vi "Demo.vi"(0 "LED Outputs":T4, 1 "VISA resource name":refnum<visa-resource-name>="COM5", 2 "Stop":bool) -> (14 "Analog Inputs":T2, 15 "Switch Inputs":T3, 16 "Updates / Second":dbl, 17 "CRC Status":bool, 18 "CRC Failures":i32)   [LabVIEW 2014]
uses:
  LED_Output_TypeDef.ctl
  Switch_Input_TypeDef.ctl
  Analog_Input_TypeDef.ctl
  PWM_Output_TypeDef.ctl
panel:
  in  "PWM Outputs":T1
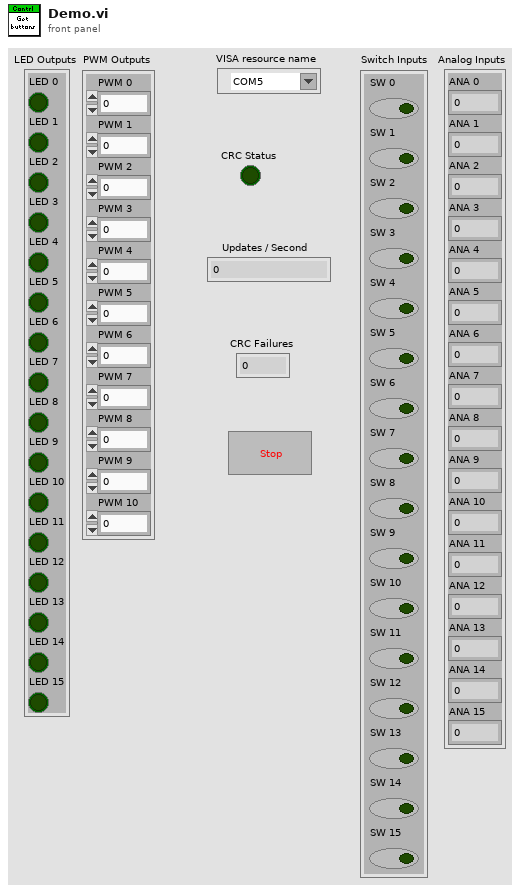
[diagram p1: front panel]
types:
  T1 = typedef "PWM_Output_TypeDef.ctl" = cluster{"PWM 0":u8, "PWM 1":u8, "PWM 2":u8, "PWM 3":u8, "PWM 4":u8, "PWM 5":u8, "PWM 6":u8, "PWM 7":u8, "PWM 8":u8, "PWM 9":u8, "PWM 10":u8}
  T2 = typedef "Analog_Input_TypeDef.ctl" = cluster{"ANA 0":u8, "ANA 1":u8, "ANA 2":u8, "ANA 3":u8, "ANA 4":u8, "ANA 5":u8, "ANA 6":u8, "ANA 7":u8, "ANA 8":u8, "ANA 9":u8, "ANA 10":u8, "ANA 11":u8, "ANA 12":u8, "ANA 13":u8, "ANA 14":u8, "ANA 15":u8}
  T3 = typedef "Switch_Input_TypeDef.ctl" = cluster{"SW 0":bool, "SW 1":bool, "SW 2":bool, "SW 3":bool, "SW 4":bool, "SW 5":bool, "SW 6":bool, "SW 7":bool, "SW 8":bool, "SW 9":bool, "SW 10":bool, "SW 11":bool, "SW 12":bool, "SW 13":bool, "SW 14":bool, "SW 15":bool}
  T4 = typedef "LED_Output_TypeDef.ctl" = cluster{"LED 0":bool, "LED 1":bool, "LED 2":bool, "LED 3":bool, "LED 4":bool, "LED 5":bool, "LED 6":bool, "LED 7":bool, "LED 8":bool, "LED 9":bool, "LED 10":bool, "LED 11":bool, "LED 12":bool, "LED 13":bool, "LED 14":bool, "LED 15":bool}
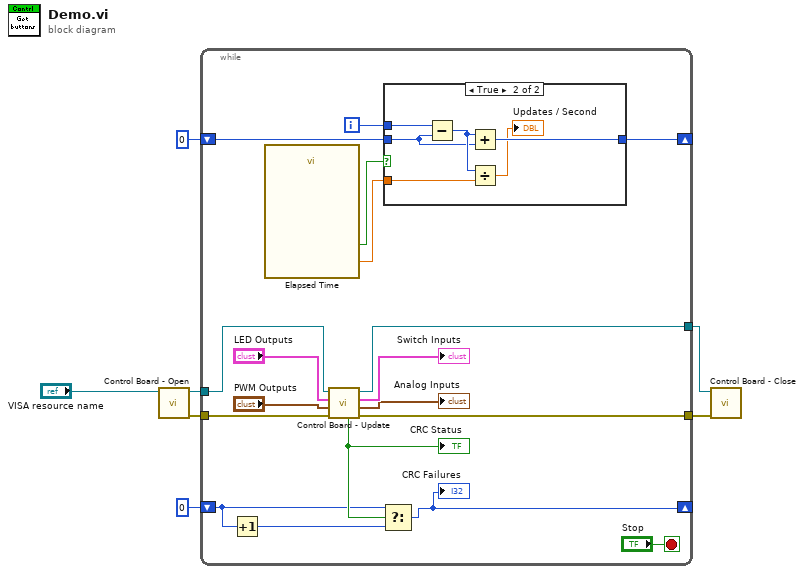
[diagram p0: block diagram]
diagram:
  n1 = call "Control Board - Open.vi"("VISA Refnum in"="VISA resource name") -> ("error out"=w2:errorcluster, "VISA Refnum out"=w3:refnum<visa-resource-name>)  [unwired: 9 in]
  n2 = while {
    tunnel: w3 -> [w24]
    tunnel: w2 -> [w23]
    tunnel: [w22] -> w7
    tunnel: [w21] -> w6
    shift-right: [w17] -> _
    shift-left: 0 -> [w18]
    shift-right: [w12] -> _
    shift-left: 0 -> [w13]
    i -> [w16]
    stop <- "Stop" stop-if-true
    n3 = Increment(x=w13) -> (x+1=w14:i32)
    n4 = call "Elapsed Time"() -> ("Elapsed Time (s)"=w19:dbl, "Time has Elapsed"=w20:bool)  [unwired: 12 in, 6 out]
    n5 = call "Control Board - Update.vi"("error in (no error)"=w23, "PWM Outputs"="PWM Outputs", "LED Outputs"="LED Outputs", "Control Board VISA Reference In"=w24) -> ("error out"=w22:errorcluster, "Analog Inputs"=→"Analog Inputs":T2, "Switch Inputs"=→"Switch Inputs":T3, "Control Board VISA Reference Out"=w21:refnum<visa-resource-name>, "CRC Status"=w15:bool)  [unwired: 3 in]
    "CRC Status" <- w15
    n6 = Select(t=w13, s=w15, f=w14) -> (s? t:f=w12:i32)
    "CRC Failures" <- w12
    n7 = case shown="True" w20 {
      tunnel: w19 -> [_ w32]
      tunnel: w18 -> [w26 w27]
      tunnel: [w26 w30] -> w17
      tunnel: w16 -> [_ w31]
      frame False {
      }
      frame True {
        n8 = Subtract(x=w31, y=w27) -> (x-y=w28:i32)
        n9 = Add(x=w28, y=w27) -> (x+y=w30:i32)
        n10 = Divide(x=w28, y=w32) -> (x/y=→"Updates / Second":dbl)
      }
    }
  }
  n11 = call "Control Board - Close.vi"("error in (no error)"=w7, "VISA Refnum in"=w6) -> ()  [unwired: 10 in]
